vi "Compare VIP PK numbers.vi"(9 "delimiter (.)":string=".", 10 "Y (#.#.#.#)":string, 11 "X (#.#.#.#)":string) -> (2 "Largest":string, 3 "X>Y":bool)   [LabVIEW 2017, in "CL_G3_VIPMUtilities.lvlib"]
doc: "Compares delimited numbers to see which is greater. Specifically used for Release.Major.Minor.Build VIP number schem. If the numbers are shaped differently, the mismatched size is padded with 0s. Examples 1.2.5 is greater than 1.2. And 2.4.3.10 is greater than 2.4.3. And 2.7.9 is less than 2.8.100."
uses:
  CL_G3_VIPMUtilities.lvlib
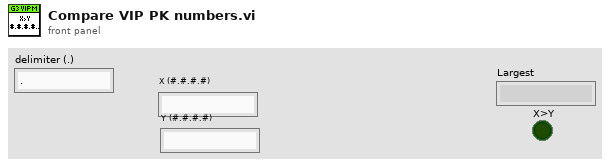
[diagram p1: front panel]
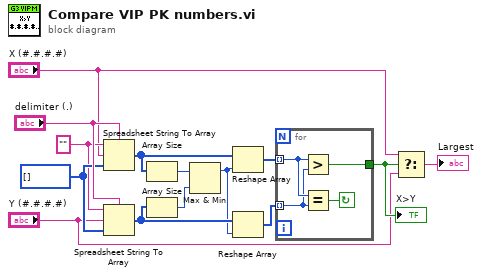
[diagram p0: block diagram]
diagram:
  w12 = "" ("format string")
  w13 = u32[] []
  n1 = Spreadsheet String To Array(delimiter (Tab)="delimiter (.)", format string=w12, spreadsheet string="X (#.#.#.#)", array type (2D Dbl)=w13) -> (array=w9:u32[])
  n2 = Spreadsheet String To Array(delimiter (Tab)="delimiter (.)", format string=w12, spreadsheet string="Y (#.#.#.#)", array type (2D Dbl)=w13) -> (array=w7:u32[])
  n3 = Array Size(array=w9) -> (size(s)=w11:i32)
  n4 = Array Size(array=w7) -> (size(s)=w10:i32)
  n5 = Max & Min(x=w11, y=w10) -> (max(x,y)=w5:i32)  [unwired: 1 out]
  n6 = Reshape Array(w9, w5) -> (w8:u32[])
  n7 = Reshape Array(w7, w5) -> (w6:u32[])
  n8 = for {
    tunnel: w8 -> [w17] mode=indexing
    tunnel: w6 -> [w16] mode=indexing
    tunnel: [w15] -> w4
    stop <- w18 continue-if-true
    n9 = Greater?(x=w17, y=w16) -> (0:w15:bool)
    n10 = Equal?(x=w17, y=w16) -> (x = y?=w18:bool)
  }
  "X>Y" <- w4
  n11 = Select(t="X (#.#.#.#)", s=w4, f="Y (#.#.#.#)") -> (s? t:f=→"Largest":string)
